vi "Method.vi"(4 "Value":refnum<class "Abs_U8 Integer.lvclass">) -> (1 "Result":refnum<class "Abs_U8 Integer.lvclass">)   [LabVIEW 2021, in "Decrement_U8.lvclass"]
uses:
  Decrement_U8.lvclass
  Abs_Types/U8 Integer/Abs_U8 Integer.lvclass
  C:/TSA/LV_Abstract/Source/Functions/Support/Function/One Terminal/U8/AbsFunc_One Term_U8.lvclass
  C:/Program Files (x86)/National Instruments/LabVIEW 2021/vi.lib/TSA/Abstract Data Classes/Abs_Types/U8 Integer/Abs_U8 Integer.lvclass
  Support/Function/One Terminal/U8/AbsFunc_One Term_U8.lvclass/AbsFunc_One Term_U8.ctl
  Support/Function/One Terminal/U8/Properties/Write Numeric A.vi
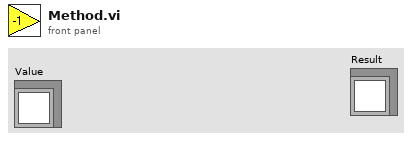
[diagram p1: front panel]
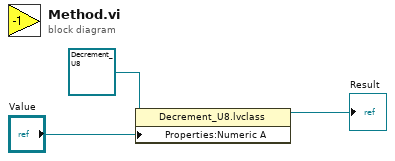
[diagram p0: block diagram]
diagram:
  n1 = property class="Decrement_U8.lvclass"(reference=refnum<class "Decrement_U8.lvclass"> refnum ("Decrement_DBL.lvclass"), "Properties:Numeric A"="Value") -> (reference out=→"Result":refnum<class "Decrement_U8.lvclass">)  [unwired: 1 in, 1 out]
